vi "voltsToCounts.vi"(8 "error in (no error)":errorcluster, 10 "Voltage":dbl[unit], 11 "VoltageToILCDACRaw in":refnum<class "VoltageToILCDACRaw.lvclass">) -> (0 "error out":errorcluster, 2 "DAC Counts":u16, 3 "VoltageToILCDACRaw out":refnum<class "VoltageToILCDACRaw.lvclass">)   [LabVIEW 2015, in "VoltageToILCDACRaw.lvclass"]
uses:
  VoltageToILCDACRaw.lvclass
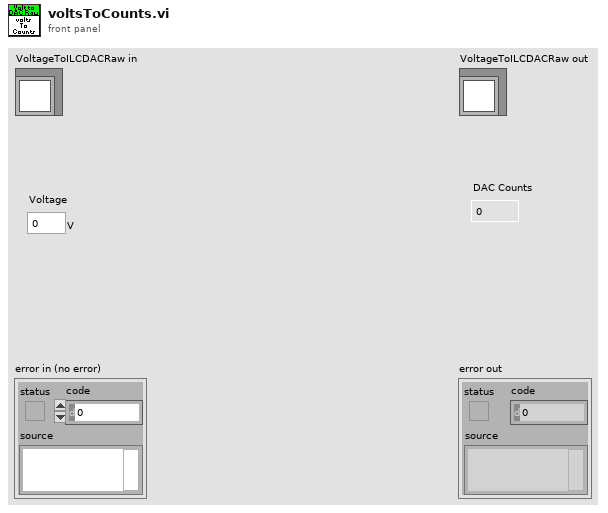
[diagram p1: front panel]
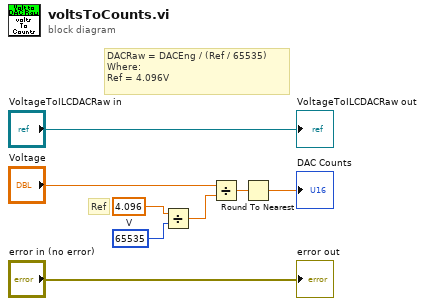
[diagram p0: block diagram]
diagram:
  w8 = dbl[unit] 4.096  # V
  # "Ref"
  # "DACRaw = DACEng / (Ref / 65535)\nWhere:\nRef = 4.096V"
  n1 = Divide(x=w8, y=65535) -> (x/y=w6:dbl[unit])
  n2 = Divide(x="Voltage", y=w6) -> (x/y=w4:dbl)
  n3 = Round To Nearest(number=w4) -> (nearest integer value=→"DAC Counts":dbl)
  "error out" <- "error in (no error)"
  "VoltageToILCDACRaw out" <- "VoltageToILCDACRaw in"
